vi "Remove Section Item By Reference.vi"(8 "error in (no error)":errorcluster, 9 "AutoDisposeSubItems(T)":bool=TRUE, 10 "Item Reference":u64 format="%.0x", 11 "Section Reference in":u64 format="%.0x") -> (0 "error out":errorcluster, 3 "Section Reference out":u64 format="%.0x", 4 "success?":bool)   [LabVIEW 2013, in "Hierarchy Framework.lvlib" / "Section.lvclass"]
doc: "Searches for <B>Item Reference</B> in the section specified by <B>Section Reference in</B> and, if found, remove and dispose the item from parent <B>Section Reference in</B> ."
uses:
  Section.lvclass
  Generic/Generic.lvclass
  Item/Item.lvclass
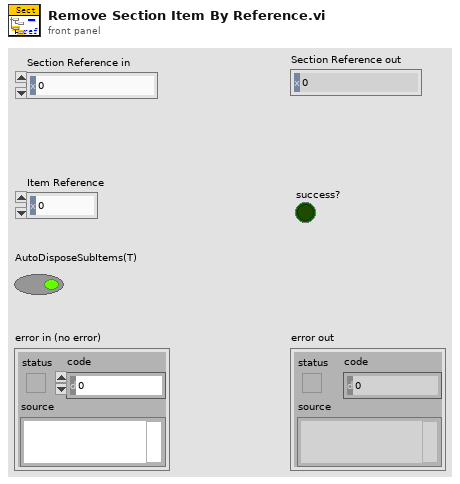
[diagram p1: front panel]
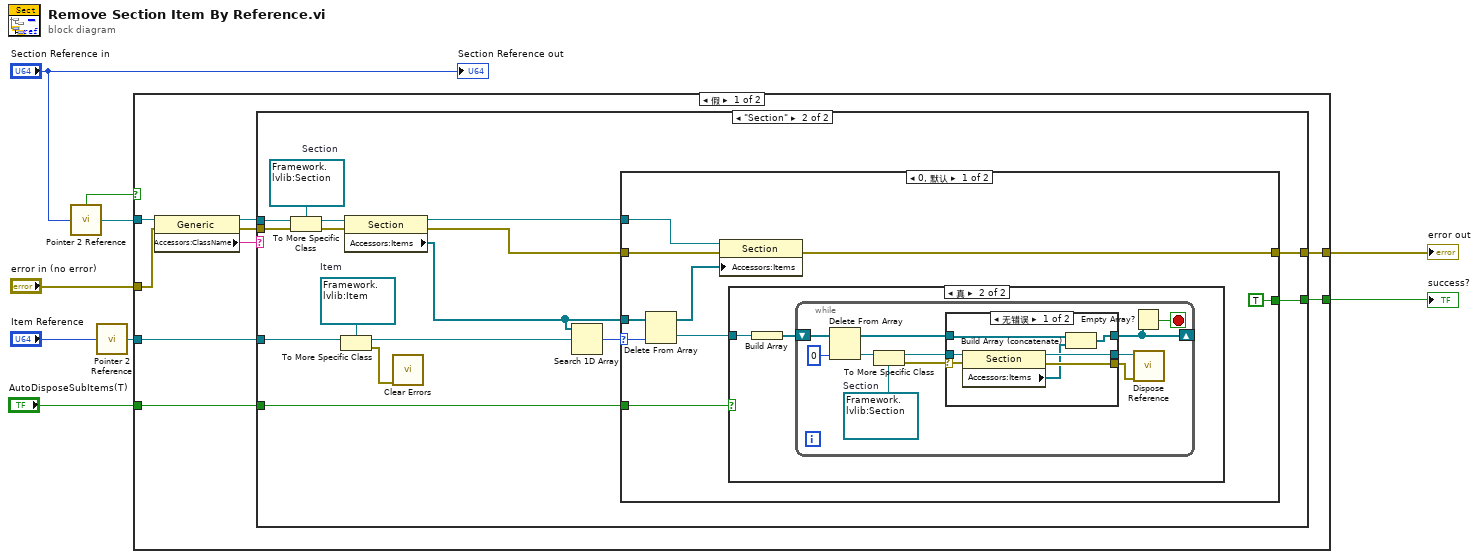
[diagram p0: block diagram]
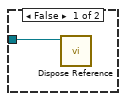
[diagram p3: hidden frame]
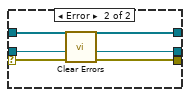
[diagram p4: hidden frame]
diagram:
  n1 = call "Pointer 2 Reference.vi"("Pointer"="Section Reference in") -> ("Not A Refnum?"=w6:bool, "Generic Reference"=w5:refnum<data-value>)
  n2 = call "Pointer 2 Reference.vi"("Pointer"="Item Reference") -> ("Generic Reference"=w2:refnum<data-value>)  [unwired: 1 out]
  n3 = case shown="假" w6 {
    tunnel: w5 -> [w17 _]
    tunnel: "error in (no error)" -> [w16 w71]
    tunnel: [w18 w71] -> w8
    tunnel: [w12 _] -> w4
    tunnel: w2 -> [w11 _]
    tunnel: "AutoDisposeSubItems(T)" -> [w10 _]
    frame False {
      n4 = property class="Generic"(reference=w17, error in=w16) -> (reference out=w14:refnum<data-value>, error out=w15:errorcluster, "Accessors:ClassName"=w13:string)
      n5 = case shown="\"Section\"" w13 {
        tunnel: [w19 w27] -> w18
        tunnel: w15 -> [w19 w32]
        tunnel: w14 -> [_ w31]
        tunnel: [_ w29] -> w12
        tunnel: w11 -> [_ w24]
        tunnel: w10 -> [_ w20]
        frame Default {
        }
        frame "Section" {
          w23 = refnum<data-value> refnum  # Item
          w35 = refnum<data-value> refnum  # Section
          n6 = To More Specific Class(target class=w35, reference=w31, error in=w32) -> (specific class reference=w34:refnum<data-value>, error out=w33:errorcluster)
          n7 = To More Specific Class(target class=w23, reference=w24) -> (specific class reference=w22:refnum<data-value>, error out=w21:errorcluster)  [unwired: 1 in]
          n8 = property class="Section"(reference=w34, error in=w33) -> (reference out=w28:refnum<data-value>, error out=w26:errorcluster, "Accessors:Items"=w25:refnum<data-value>[])
          n9 = call <vilib>:"Clear Errors.vi"("error in (no error)"=w21) -> ()  [unwired: 6 in, 1 out]
          n10 = Search 1D Array(1D array=w25, element=w22) -> (index of element=w30:i32)  [unwired: 1 in]
          n11 = case shown="0, 默认" w30 {
            selector: w30 -> [w44 _]
            tunnel: w25 -> [w43 _]
            tunnel: [TRUE _] -> w29
            tunnel: w28 -> [w41 _]
            tunnel: w26 -> [w39 w70]
            tunnel: [w38 w70] -> w27
            tunnel: w20 -> [w36 _]
            frame 0, Default {
              n12 = Delete From Array(array=w43, index=w44) -> (deleted portion=w37:refnum<data-value>, array with subset deleted=w40:refnum<data-value>[])  [unwired: 1 in]
              n13 = property class="Section"(reference=w41, error in=w39, "Accessors:Items"=w40) -> (error out=w38:errorcluster)  [unwired: 1 out]
              n14 = case shown="真" w36 {
                tunnel: w37 -> [w45 w47]
                frame False {
                  n15 = call "Dispose Reference.vi"("Generic Reference"=w45) -> ()  [unwired: 10 in, 1 out]
                }
                frame True {
                  n16 = Build Array(w47) -> (w46:refnum<data-value>[])
                  n17 = while {
                    shift-right: [w49] -> _
                    shift-left: w46 -> [w58]
                    stop <- w48 stop-if-true
                    w55 = refnum<data-value> refnum  # Section
                    n18 = Delete From Array(array=w58, index=0 ("索引")) -> (deleted portion=w56:refnum<data-value>, array with subset deleted=w52:refnum<data-value>[])  [unwired: 1 in]
                    n19 = To More Specific Class(target class=w55, reference=w56) -> (specific class reference=w53:refnum<data-value>, error out=w54:errorcluster)  [unwired: 1 in]
                    n20 = case shown="无错误" w54 {
                      selector: w54 -> [w65 w67]
                      tunnel: w53 -> [w64 w68]
                      tunnel: w52 -> [w63 w69]
                      tunnel: [w62 w69] -> w49
                      tunnel: [w61 w68] -> w51
                      tunnel: [w60 w66] -> w50
                      frame No Error {
                        n21 = property class="Section"(reference=w64, error in=w65) -> (reference out=w61:refnum<data-value>, error out=w60:errorcluster, "Accessors:Items"=w59:refnum<data-value>[])
                        n22 = Build Array (concatenate)(w63, w59) -> (w62:refnum<data-value>[])
                      }
                      frame Error {
                        n23 = call <vilib>:"Clear Errors.vi"("error in (no error)"=w67) -> ("error out"=w66:errorcluster)  [unwired: 6 in]
                      }
                    }
                    n24 = Empty Array?(array=w49) -> (empty?=w48:bool)
                    n25 = call "Dispose Reference.vi"("error in (no error)"=w50, "Generic Reference"=w51) -> ()  [unwired: 9 in, 1 out]
                  }
                }
              }
            }
            frame -1 {
            }
          }
        }
      }
    }
    frame True {
    }
  }
  "error out" <- w8
  "success?" <- w4
  "Section Reference out" <- "Section Reference in"
